vi "cal sensor buffer.vi"(4 "command":T3, 5 "smooth interval (s)":sgl format="%.3f", 6 "max array size":u16=1 min=1, 7 "Sensor Data":T1 {"Sensor array"."scaled" format="%.2f"; "Sensor array"."voltage" format="%.4f"; "Time" format="%<%I:%M:%S%2u %p\n%m/%d/%Y>T"}) -> (1 "data rate (Hz)":sgl format="%.2f", 2 "all sensor data":T1[](array[typedef]) {"Sensor array"."scaled" format="%.2f"; "Sensor array"."voltage" format="%.4f"; "Time" format="%<%I:%M:%S%2u %p\n%m/%d/%Y>T"}, 3 "Sensor Data smoothed":T1 {"Sensor array"."scaled" format="%.2f"; "Sensor array"."voltage" format="%.4f"; "Time" format="%<%I:%M:%S%2u %p\n%m/%d/%Y>T"})   [LabVIEW 2012]
doc: "Sensor buffer stores sensor data in an array. \nThe buffer must be configured using the configure command and must be given the maximum array size\n\nNew data is added to the buffer using the write command.\n\nAverage data from the last \"smooth interval\" seconds can be accessed using the average command.\n\nThe most recent data can be accessed using the recent command.\n\nThe data is arranged with the newest data at index 0."
uses:
  TCP DAQ/Sensor data.ctl
  DAQ configuration/sensor cluster.ctl
  DAQ configuration/Sensor buffer command.ctl
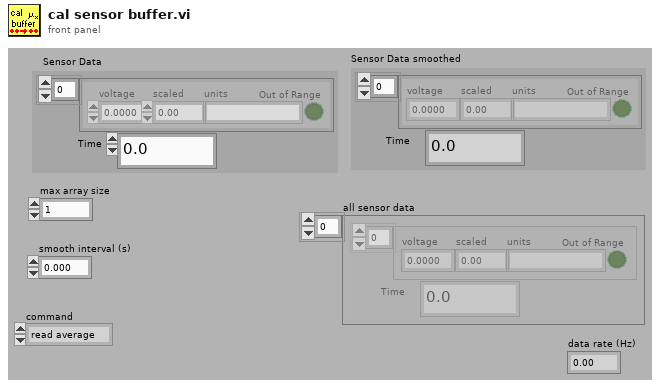
[diagram p1: front panel]
types:
  T1 = typedef "Sensor data.ctl" = cluster{" Sensor array":T2[], "Time":dbl}
  T2 = typedef "sensor cluster.ctl" = cluster{"voltage":sgl, "scaled":sgl, "units":string, "Out of Range":bool}
  T3 = typedef "Sensor buffer command.ctl" = enum16{"read average", "read recent", "read all", "write", "configure", "clear"}
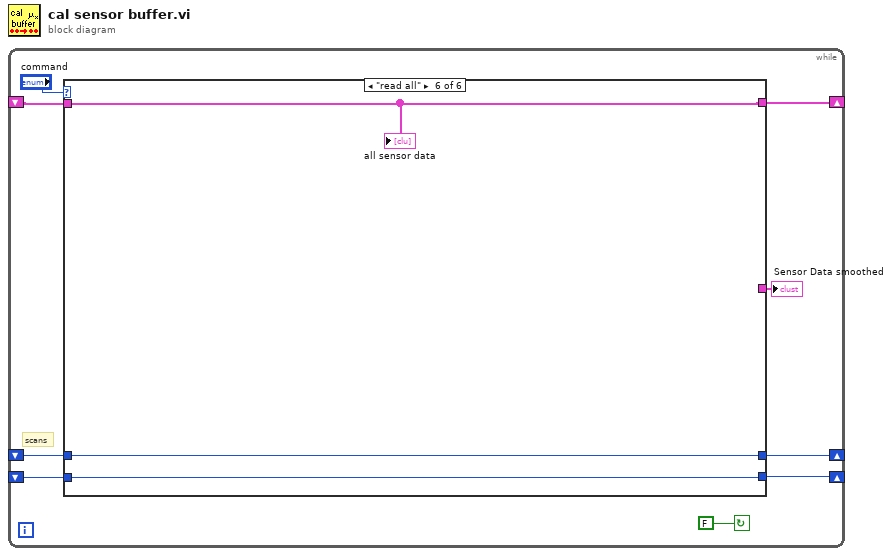
[diagram p0: block diagram]
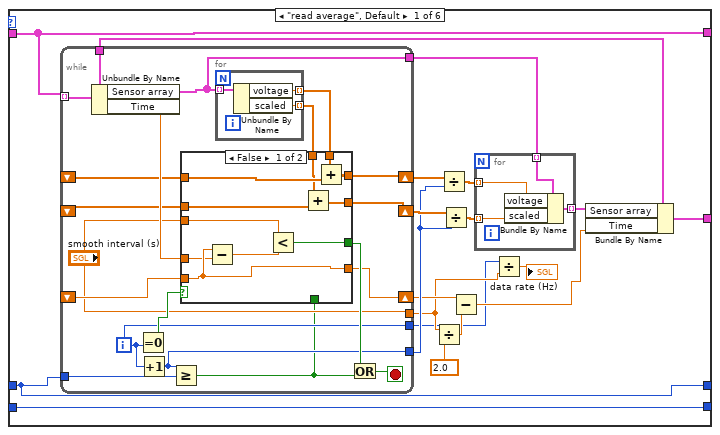
[diagram p2: hidden frame]
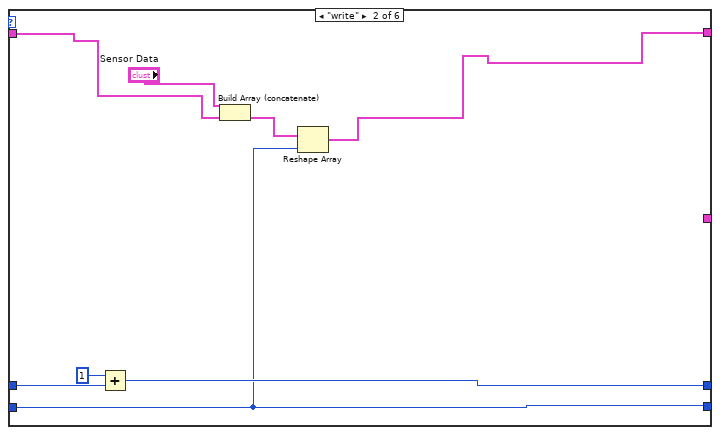
[diagram p4: hidden frame]
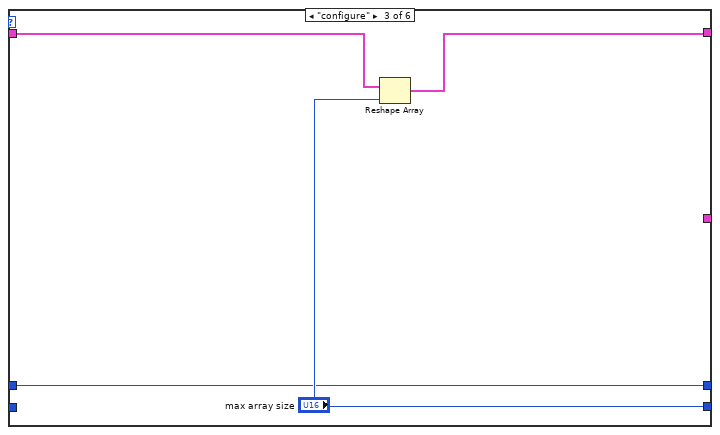
[diagram p5: hidden frame]
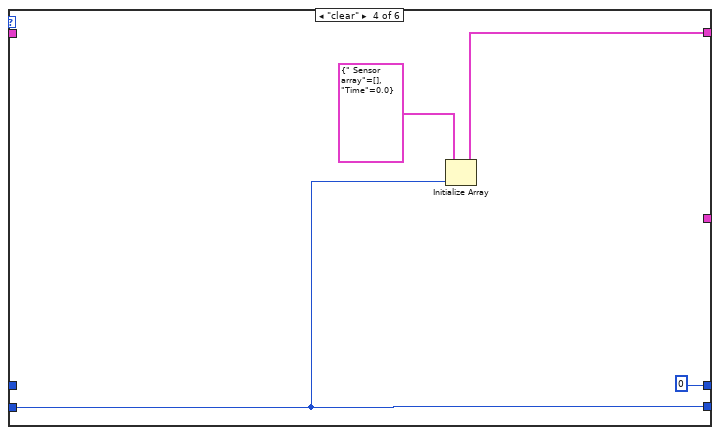
[diagram p6: hidden frame]
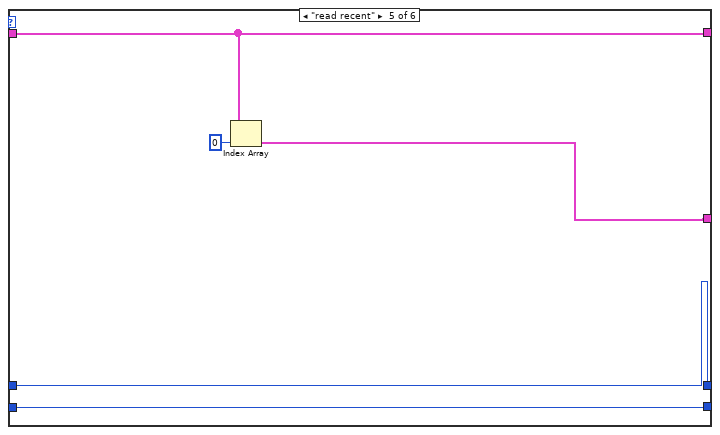
[diagram p7: hidden frame]
diagram:
  n1 = while {
    shift-right: [w8] -> _
    shift-left: _ -> [w7]
    shift-right: [w6] -> _
    shift-left: _ -> [w5]
    shift-right: [w1] -> _
    shift-left: _ -> [w2]
    stop <- FALSE continue-if-true
    # "scans"
    n2 = case shown="\"read all\"" "command" {
      tunnel: [w14 w71 w80 w84 w90 w93] -> w8
      tunnel: w7 -> [w14 w75 w79 _ w90 w93]
      tunnel: [w28 w72 "max array size" w83 w87 w92] -> w6
      tunnel: w5 -> [w28 w72 _ w83 w87 w92]
      tunnel: [w19 _ _ _ w88 _] -> w3
      tunnel: w2 -> [w13 w73 w78 _ w86 w91]
      tunnel: [w13 w76 w78 0 w86 w91] -> w1
      frame "read average", Default {
        n3 = while {
          tunnel: w14 -> [w36] mode=indexing
          shift-right: [w35] -> w24
          shift-left: _ -> [w50]
          tunnel: w13 -> [w46]
          shift-right: [w43] -> w27
          shift-left: _ -> [w41]
          shift-right: [w42] -> w26
          shift-left: _ -> [w40]
          tunnel: [w37] -> w25
          tunnel: ["smooth interval (s)"] -> w12
          tunnel: [w36] -> w18
          tunnel: [w33] -> w15
          tunnel: [w38] -> w10
          i -> [w38]
          stop <- w47 stop-if-true
          n4 = Unbundle By Name(w36) -> ("Sensor array"=w33:T2[], "Time"=w51:dbl)
          n5 = Equal To 0?(x=w38) -> (x = 0?=w49:bool)
          n6 = Increment(x=w38) -> (x+1=w37:i32)
          n7 = Greater Or Equal?(x=w37, y=w46) -> (x >= y?=w34:bool)
          n8 = for {
            tunnel: w33 -> [w67] mode=indexing
            tunnel: [w69] -> w45 mode=indexing
            tunnel: [w68] -> w44 mode=indexing
            n9 = Unbundle By Name(w67) -> ("voltage"=w69:sgl, "scaled"=w68:sgl)
          }
          n10 = case shown="False" w49 {
            tunnel: w51 -> [w52 w66]
            tunnel: [w53 w66] -> w35
            tunnel: w50 -> [w53 _]
            tunnel: [w61 w63] -> w48
            tunnel: [w58 w65] -> w43
            tunnel: w45 -> [w60 w65]
            tunnel: [w57 w64] -> w42
            tunnel: w44 -> [w56 w64]
            tunnel: w41 -> [w59 _]
            tunnel: w40 -> [w55 _]
            tunnel: "smooth interval (s)" -> [w54 _]
            tunnel: w34 -> [_ w63]
            frame False {
              n11 = Subtract(x=w53, y=w52) -> (x-y=w62:dbl)
              n12 = Less?(x=w54, y=w62) -> (x < y?=w61:bool)
              n13 = Add(x=w56, y=w55) -> (x+y=w57:sgl[])
              n14 = Add(x=w60, y=w59) -> (x+y=w58:sgl[])
            }
            frame True {
            }
          }
          n15 = Or(x=w48, y=w34) -> (x .or. y?=w47:bool)
        }
        n16 = Divide(x=w12, y=sgl 2.0) -> (x/y=w22:sgl)
        n17 = Divide(x=w27, y=w25) -> (x/y=w21:sgl[])
        n18 = Divide(x=w26, y=w25) -> (x/y=w20:sgl[])
        n19 = Subtract(x=w24, y=w22) -> (x-y=w16:dbl)
        n20 = for {
          tunnel: w15 -> [w32] mode=indexing
          tunnel: w21 -> [w31] mode=indexing
          tunnel: w20 -> [w30] mode=indexing
          tunnel: [w29] -> w17 mode=indexing
          n21 = Bundle By Name(cluster=w32, "voltage"=w31, "scaled"=w30) -> (w29:T2)
        }
        n22 = Divide(x=w10, y=w12) -> (x/y=→"data rate (Hz)":sgl)
        n23 = Bundle By Name(cluster=w18, "Sensor array"=w17, "Time"=w16) -> (w19:T1)
      }
      frame "write" {
        n24 = Add(x=1, y=w73) -> (x+y=w76:i32)
        n25 = Build Array (concatenate)("Sensor Data", w75) -> (w70:T1[])
        n26 = Reshape Array(w70, w72) -> (w71:T1[])
      }
      frame "configure" {
        n27 = Reshape Array(w79, "max array size") -> (w80:T1[])
      }
      frame "clear" {
        n28 = Initialize Array(T1 {" Sensor array"=[], "Time"=0.0} ("Sensor Data"), w83) -> (w84:T1[])
      }
      frame "read recent" {
        n29 = Index Array(array=w90, index=0) -> (element=w88:T1)
      }
      frame "read all" {
        "all sensor data" <- w93
      }
    }
    "Sensor Data smoothed" <- w3
  }
